vi "errorHandlerDLL.vi"(7 "show popup":bool, 9 "language":i32, 10 "error number":i8, 11 "connection ID":i32) -> (0 "error out":errorcluster, 3 "connection ID":i32)   [LabVIEW 2016]
panel:
  in  "error in":errorcluster
  in  "results cluster":cluster{"errNo":i32, "result":string}
  out "params_cluster":cluster{"params":i64, "language":i64}
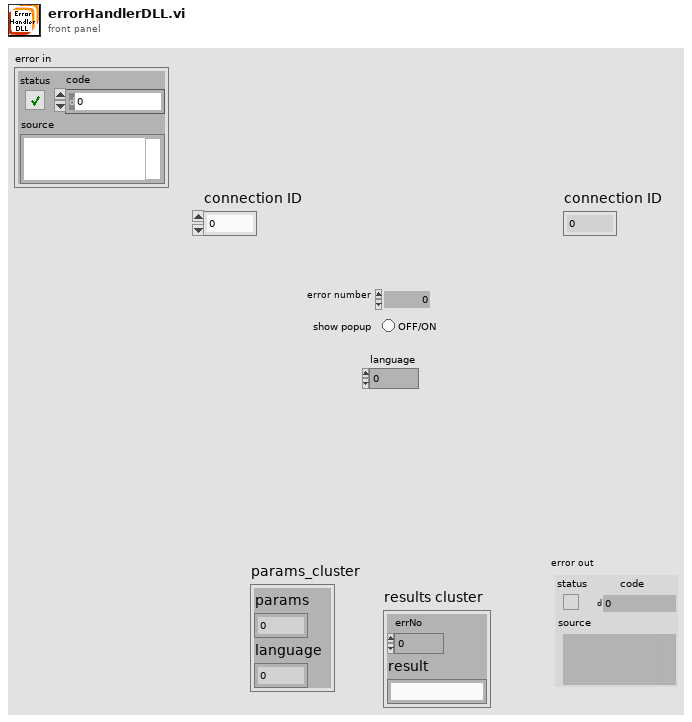
[diagram p1: front panel]
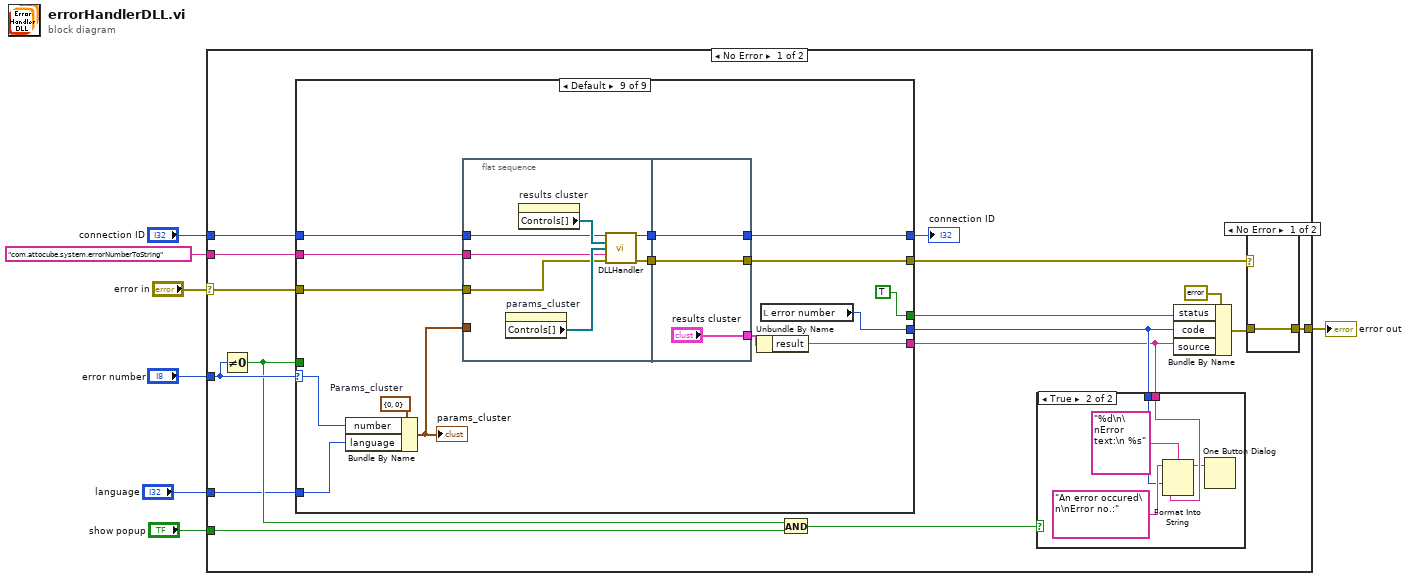
[diagram p0: block diagram]
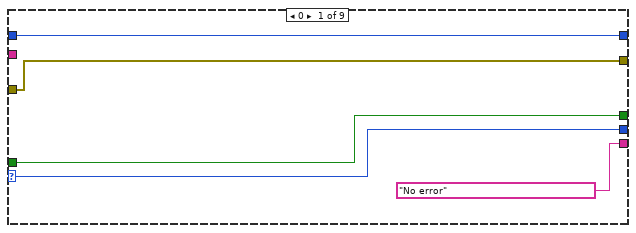
[diagram p4: hidden frame]
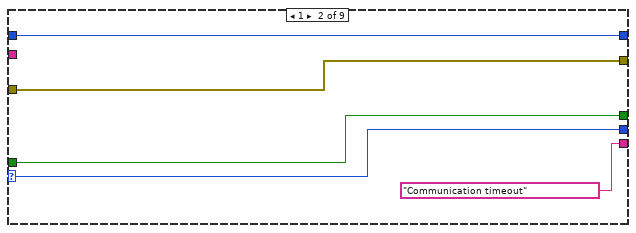
[diagram p5: hidden frame]
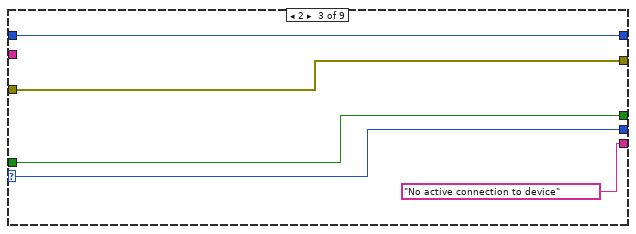
[diagram p6: hidden frame]
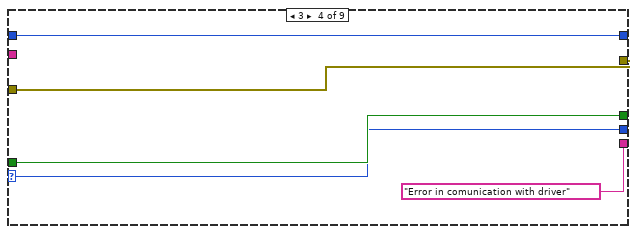
[diagram p7: hidden frame]
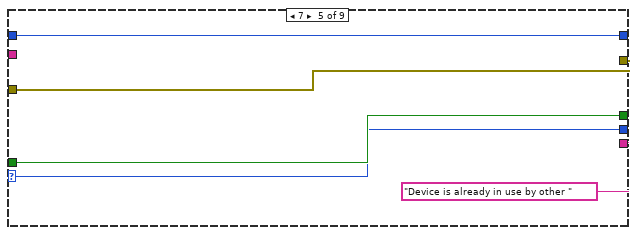
[diagram p8: hidden frame]
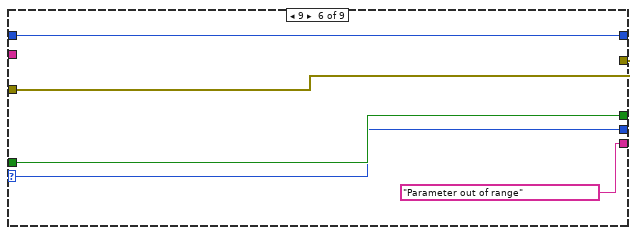
[diagram p9: hidden frame]
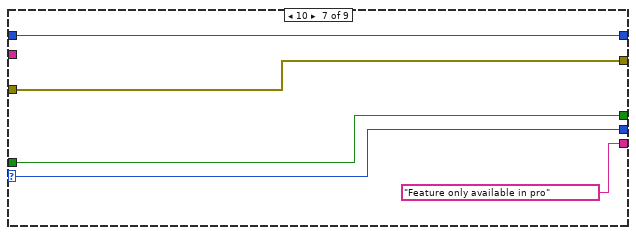
[diagram p10: hidden frame]
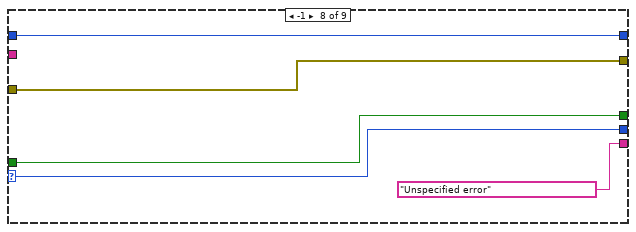
[diagram p11: hidden frame]
diagram:
  n1 = case shown="No Error" "error in" {
    selector: "error in" -> [w8 w96]
    tunnel: "error number" -> [w23 _]
    tunnel: "show popup" -> [w18 _]
    tunnel: "language" -> [w16 _]
    tunnel: "connection ID" -> [w13 _]
    tunnel: "com.attocube.system.errorNumberToString" ("Set Command") -> [w12 _]
    tunnel: [w9 w96] -> w2
    frame No Error {
      n2 = Not Equal To 0?(x=w23) -> (x != 0?=w19:bool)
      n3 = case shown="Default" w23 {
        selector: w23 -> [w34 w40 w44 w49 w54 w59 w64 w69 w80]
        tunnel: ["No error" "Communication timeout" "No active connection to device" "Error in comunication with driver" "Device is already in use by other " "Parameter out of range" "Feature only available in pro" "Unspecified error" w75] -> w20
        tunnel: [w34 w40 w44 w49 w54 w59 w64 w69 w71] -> w21
        tunnel: [w33 w39 w43 w50 w55 w60 w63 w70 TRUE] -> w22
        tunnel: w19 -> [w33 w39 w43 w50 w55 w60 w63 w70 _]
        tunnel: w16 -> [_ _ _ _ _ _ _ _ w81]
        tunnel: [w32 w37 w42 w47 w52 w57 w62 w67 w83] -> w14
        tunnel: w13 -> [w32 w37 w42 w47 w52 w57 w62 w67 w82]
        tunnel: w12 -> [_ _ _ _ _ _ _ _ w79]
        tunnel: w8 -> [w31 w36 w41 w46 w51 w56 w61 w66 w78]
        tunnel: [w31 w36 w41 w46 w51 w56 w61 w66 w73] -> w11
        frame 0 {
        }
        frame 1 {
        }
        frame 2 {
        }
        frame 3 {
        }
        frame 7 {
        }
        frame 9 {
        }
        frame 10 {
        }
        frame -1 {
        }
        frame Default {
          w84 = cluster{"number":i64, "language":i64} {"number"=0, "language"=0}  # Params_cluster
          n4 = Bundle By Name(cluster=w84, "number"=w80, "language"=w81) -> (w74:cluster{"number":i64, "language":i64})
          "params_cluster" <- w74
          n5 = flat-sequence {
            tunnel: w82 -> [w89]
            tunnel: w79 -> [w88]
            tunnel: w78 -> [w87]
            tunnel: [w90] -> w77
            tunnel: w74 -> [_]
            tunnel: [w86] -> w72
            tunnel: [w95] -> w83
            tunnel: w77 -> [w95]
            tunnel: ["results cluster"] -> w76
            tunnel: [w93] -> w73
            tunnel: w72 -> [w93]
            frame #0 {
              n6 = property on="params_cluster" class="Clust (strict)"() -> ("Controls[]"=w92:refnum<vi>[])  [unwired: 2 in, 2 out]
              n7 = property on="results cluster" class="Clust (strict)"() -> ("Controls[]"=w91:refnum<vi>[])  [unwired: 2 in, 2 out]
              n8 = call "DLLHandler.vi"("connection ID"=w89, "results_cluster"=w91, "params_cluster"=w92, "method"=w88, "error"=w87) -> ("connection ID out"=w90:i32, "error"=w86:errorcluster)  [unwired: 9 in]
            }
            frame #1 {
            }
          }
          n9 = Unbundle By Name(w76) -> ("result"=w75:string)
          n10 = local read "error number"() -> (w71:i8)
        }
      }
      "connection ID" <- w14
      n11 = And(x=w19, y=w18) -> (x .and. y?=w17:bool)
      n12 = case shown="True" w17 {
        tunnel: w21 -> [_ w29]
        tunnel: w20 -> [_ w27]
        frame False {
        }
        frame True {
          n13 = Format Into String(format string="%d\n\nError text:\n %s", initial string="An error occured\n\nError no.:", w29, w27) -> (resulting string=w26:string)  [unwired: 1 in, 1 out]
          n14 = One Button Dialog(message=w26) -> ()  [unwired: 1 in, 1 out]
        }
      }
      n15 = Bundle By Name(cluster=errorcluster {"status"=FALSE, "code"=0, "source"=""} ("error in"), "status"=w22, "code"=w21, "source"=w20) -> (w10:errorcluster)
      n16 = case shown="No Error" w11 {
        selector: w11 -> [_ w25]
        tunnel: w10 -> [w24 _]
        tunnel: [w24 w25] -> w9
        frame No Error {
        }
        frame Error {
        }
      }
    }
    frame Error {
    }
  }
  "error out" <- w2
